vi "Ramp signal generation.vi"() -> ()   [LabVIEW 2020]
uses:
  <vilib>/DAQmx/write.llb/DAQmx Write (Analog DBL 1Chan 1Samp).vi
  <vilib>/Analysis/1siggen.llb/Ramp Pattern by Delta.vi
  <vilib>/DAQmx/create/channels.llb/DAQmx Create Channel (AO-Voltage-Basic).vi
  <vilib>/DAQmx/miscellaneous.llb/DAQmx Fill In Error Info.vi
  <vilib>/Analysis/NI_AALBase.lvlib
panel:
  out "samples":i32
  out "Waveform Graph 2":dbl[](graph)
  out "Waveform Graph":dbl[](graph)
  out "number of samples written per channel":u32
  out "x+y":dbl
  in  "End position (mm)":dbl
  out "Total Z thickness (mm)":dbl
  in  "Z slice width (mm)":dbl
  in  "Start position(mm)":dbl
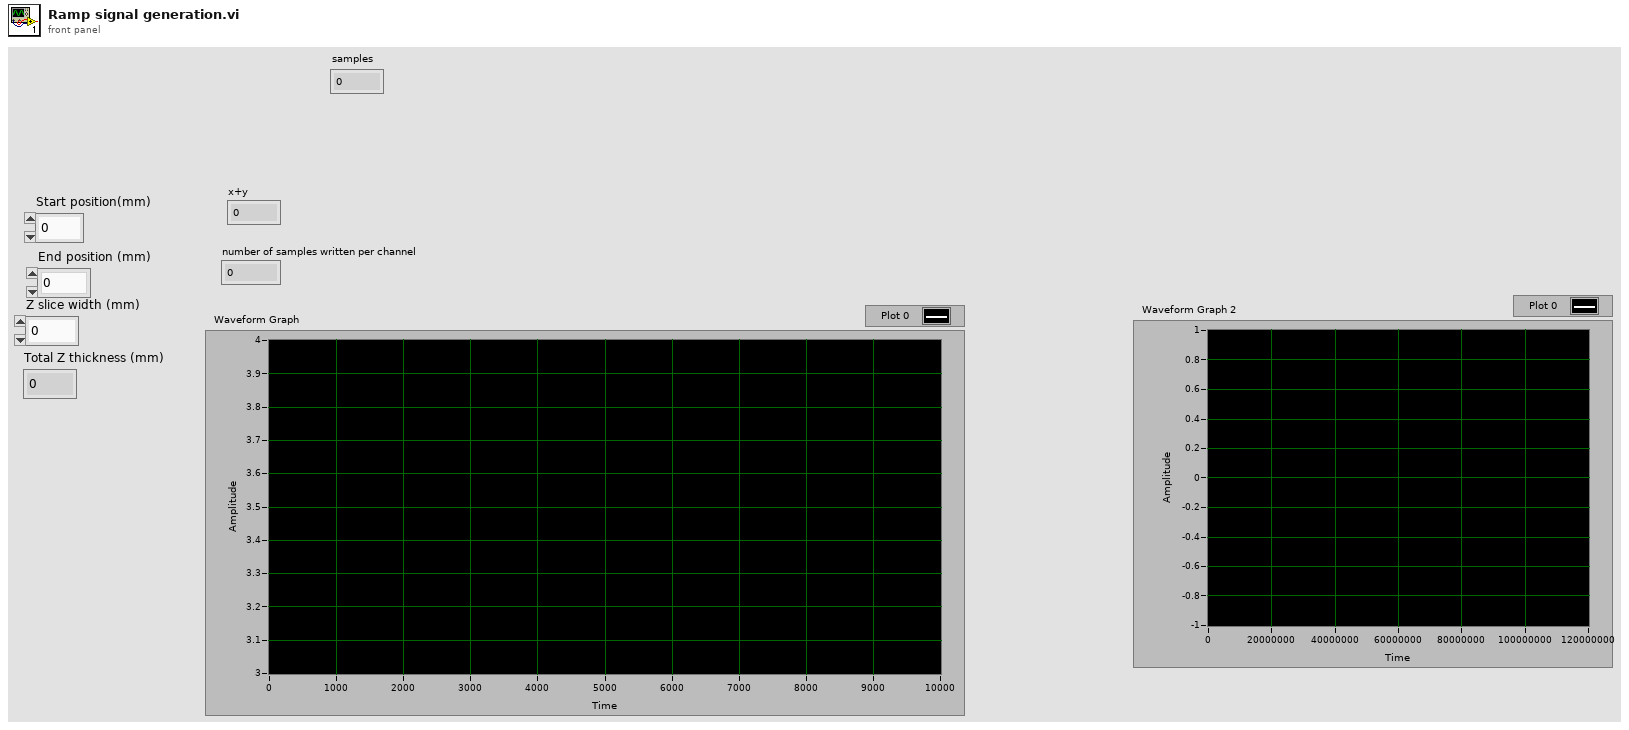
[diagram p1: front panel]
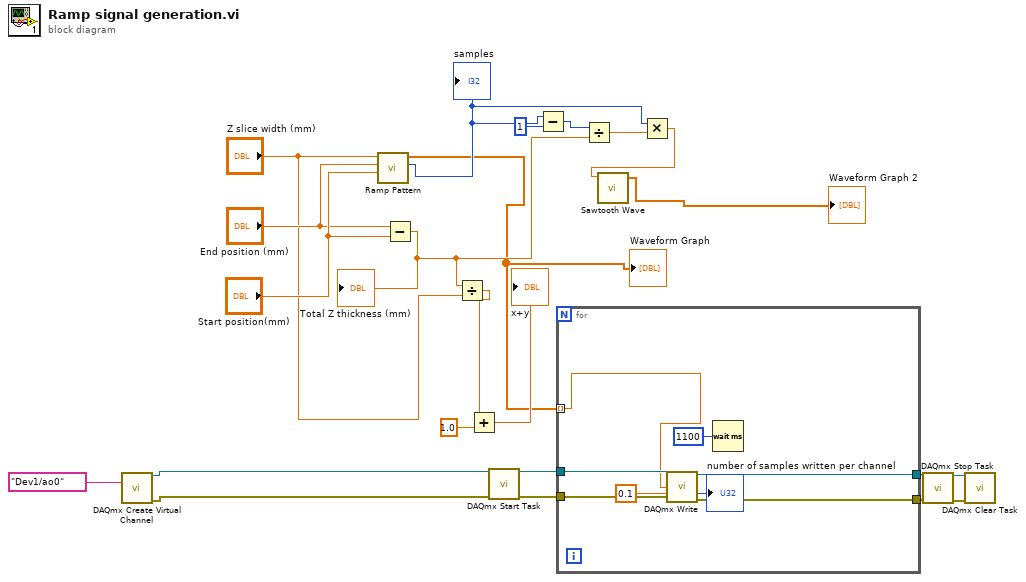
[diagram p0: block diagram]
diagram:
  n1 = call-poly <vilib>:"DAQmx Create Virtual Channel.vi"("physical channels"=tag "Dev1/ao0") -> ("task out"=w21:refnum<k21>, "error out"=w20:errorcluster)  [unwired: 13 in]
  n2 = call-poly <vilib>:"Ramp Pattern.vi"("start"="Start position(mm)", "end"="End position (mm)", "delta"="Z slice width (mm)") -> ("samples"=w4:i32, "Ramp Pattern"=w1:dbl[])  [unwired: 6 in, 1 out]
  "samples" <- w4
  "Waveform Graph" <- w1
  n3 = Subtract(x="End position (mm)", y="Start position(mm)") -> (x-y=w5:dbl)
  "Total Z thickness (mm)" <- w5
  n4 = Divide(x=w5, y="Z slice width (mm)") -> (x/y=w10:dbl)
  n5 = Add(x=w10, y=1.0) -> (x+y=→"x+y":dbl)
  n6 = call <vilib>:"DAQmx Start Task.vi"("task/channels in"=w21, "error in"=w20) -> ("task out"=w14:refnum<k21>, "error out"=w13:errorcluster)  [unwired: 12 in]
  n7 = Subtract(x=w4, y=1) -> (x-y=w6:i32)
  n8 = for {
    tunnel: [w31] -> w16
    tunnel: [w30] -> w15
    tunnel: w14 -> [w29]
    tunnel: w13 -> [w28]
    tunnel: w1 -> [w24] mode=indexing
    n9 = call-poly <vilib>:"DAQmx Write.vi"("task/channels in"=w29, "data"=w24, "timeout"=0.1, "error in"=w28) -> ("task out"=w31:refnum<k21>, "number of samples written per channel"=→"number of samples written per channel":u32, "error out"=w30:errorcluster)  [unwired: 9 in]
    n10 = Wait (ms)(milliseconds to wait=u32 1100) -> ()  [unwired: 1 out]
  }
  n11 = Divide(x=w6, y=w5) -> (x/y=w3:dbl)
  n12 = Multiply(x=w4, y=w3) -> (x*y=w2:dbl)
  n13 = call <vilib>:"Sawtooth Wave.vi"("samples"=w2) -> ("sawtooth wave"=→"Waveform Graph 2":dbl[])  [unwired: 4 in, 2 out]
  n14 = call <vilib>:"DAQmx Stop Task.vi"("task/channels in"=w16, "error in"=w15) -> ("task out"=w18:refnum<k21>, "error out"=w17:errorcluster)  [unwired: 12 in]
  n15 = call <vilib>:"DAQmx Clear Task.vi"("task in"=w18, "error in"=w17) -> ()  [unwired: 13 in, 1 out]
